vi "LTE ModAcc Fetch.vi"(0 "RFmx Handle In":refnum<k21>, 1 "Selector String":string, 11 "error in (no error)":errorcluster) -> (4 "RFmx Handle Out":refnum<k21>, 6 "ModAcc Results":T1, 15 "error out":errorcluster)   [LabVIEW 2018, in "RFmxLTE.lvlib"]
uses:
  RFmxLTE.lvlib
  Typedefs/LTE ModAcc Results.ctl
  Typedefs/LTE ModAcc CC Results.ctl
  <vilib>/RFmx/LTE/mx/RFmxLTE.llb/RFmxLTE ModAcc Fetch Composite EVM (Array).vi
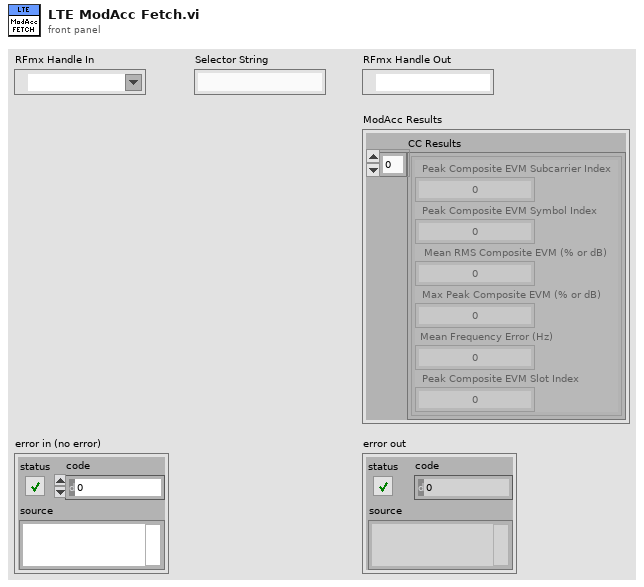
[diagram p1: front panel]
types:
  T1 = typedef "RFmxLTE.lvlib/LTE ModAcc Results.ctl" = cluster{"CC Results":T2[]}
  T2 = typedef "RFmxLTE.lvlib/LTE ModAcc CC Results.ctl" = cluster{"Peak Composite EVM Subcarrier Index":i32, "Peak Composite EVM Symbol Index":i32, "Mean RMS Composite EVM (% or dB)":dbl, "Max Peak Composite EVM (% or dB)":dbl, "Mean Frequency Error (Hz)":dbl, "Peak Composite EVM Slot Index":i32}
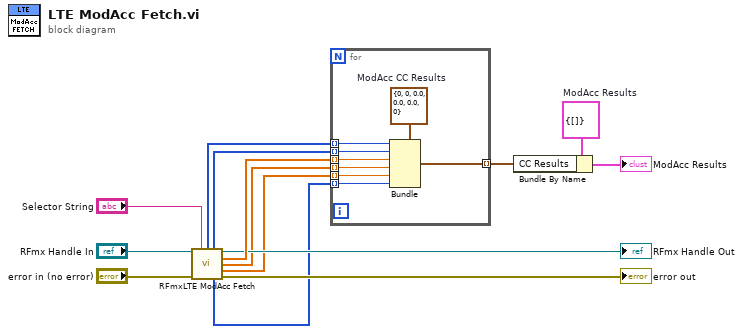
[diagram p0: block diagram]
diagram:
  w14 = T1 {"CC Results"=[]}  # ModAcc Results
  n1 = call-poly <vilib>:"RFmxLTE ModAcc Fetch.vi"("Instrument Handle In"="RFmx Handle In", "Selector String"="Selector String", "error in (no error)"="error in (no error)") -> ("Peak Composite EVM Subcarrier Index"=w8:i32[], "Peak Composite EVM Symbol Index"=w7:i32[], "Instrument Handle Out"=→"RFmx Handle Out":refnum<k21>, "Mean RMS Composite EVM (% or dB)"=w6:dbl[], "Max Peak Composite EVM (% or dB)"=w3:dbl[], "Mean Frequency Error (Hz)"=w2:dbl[], "Peak Composite EVM Slot Index"=w1:i32[], "error out"=→"error out":errorcluster)  [unwired: 5 in]
  n2 = for {
    tunnel: [w22] -> w12 mode=indexing
    tunnel: w8 -> [w20] mode=indexing
    tunnel: w7 -> [w19] mode=indexing
    tunnel: w6 -> [w18] mode=indexing
    tunnel: w3 -> [w17] mode=indexing
    tunnel: w2 -> [w16] mode=indexing
    tunnel: w1 -> [w15] mode=indexing
    w21 = T2 {"Peak Composite EVM Subcarrier Index"=0, "Peak Composite EVM Symbol Index"=0, "Mean RMS Composite EVM (% or dB)"=0.0, "Max Peak Composite EVM (% or dB)"=0.0, "Mean Frequency Error (Hz)"=0.0, "Peak Composite EVM Slot Index"=0}  # ModAcc CC Results
    n3 = Bundle(cluster=w21, "Peak Composite EVM Subcarrier Index"=w20, "Peak Composite EVM Symbol Index"=w19, "Mean RMS Composite EVM (% or dB)"=w18, "Max Peak Composite EVM (% or dB)"=w17, "Mean Frequency Error (Hz)"=w16, "Peak Composite EVM Slot Index"=w15) -> (w22:T2)
  }
  n4 = Bundle By Name(cluster=w14, "CC Results"=w12) -> (→"ModAcc Results":T1)
